vi "hardcode_libs.vi"() -> ()   [LabVIEW 2019]
uses:
  <vilib>/Utility/traverseref.llb/TRef TravTarget.ctl
  <vilib>/Utility/traverseref.llb/VI Scripting - Traverse.lvlib
panel:
  out "current":string
  out "progress":i32(slide) scale=-1.0..35.0
  # "Hardcode library paths"
  # "Use this if you have problems with DLL resolution in deployed applications. Use with caution."
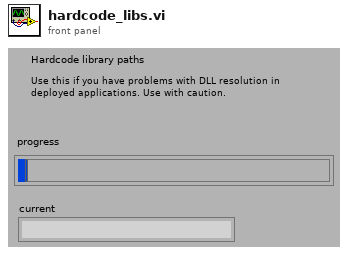
[diagram p1: front panel]
types:
  T1 = typedef "TRef TravTarget.ctl" = enum16{"FP", "BD", "Other"}
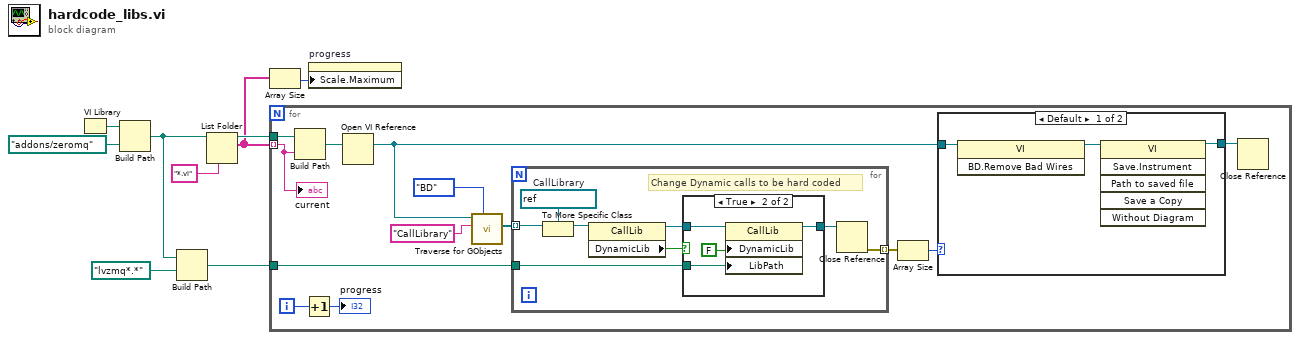
[diagram p0: block diagram]
diagram:
  n1 = VI Library() -> (path=w6:path)
  n2 = Build Path(base path=w6, name or relative path=path "addons/zeromq" ("Relative path (.)")) -> (appended path=w2:path)
  n3 = Build Path(base path=w2, name or relative path=path "lvzmq*.*" ("Library Path")) -> (appended path=w1:path)
  n4 = List Folder(path=w2, pattern="*.vi") -> (path out=w8:path, filenames=w5:string[])  [unwired: 2 in, 2 out]
  n5 = Array Size(array=w5) -> (size(s)=w4:i32)
  n6 = for {
    tunnel: w5 -> [w15] mode=indexing
    tunnel: w8 -> [w22]
    tunnel: w1 -> [w11]
    i -> [w14]
    n7 = Build Path(base path=w22, name or relative path=w15) -> (appended path=w21:path)
    n8 = Increment(x=w14) -> (x+1=→"progress":i32)
    n9 = Open VI Reference(vi path=w21) -> (vi reference=w17:refnum<vi>)  [unwired: 5 in, 1 out]
    n10 = call <vilib>:"Traverse for GObjects.vi"("Traverse Target"=TRef_TravTarget."BD", "Class Name"="CallLibrary", "VI Refnum"=w17) -> ("References"=w18:refnum<vi>[])  [unwired: 5 in, 3 out]
    n11 = for {
      tunnel: w18 -> [w34] mode=indexing
      tunnel: [w31] -> w13 mode=indexing
      tunnel: w11 -> [w30]
      w33 = refnum<vi> refnum  # CallLibrary
      # "Change Dynamic calls to be hard coded"
      n12 = To More Specific Class(target class=w33, reference=w34) -> (specific class reference=w29:refnum<vi>)  [unwired: 1 in, 1 out]
      n13 = property class="CallLib"(reference=w29) -> (reference out=w28:refnum<vi>, "DynamicLib"=w27:bool)  [unwired: 1 in, 1 out]
      n14 = case shown="True" w27 {
        tunnel: [w35 w39] -> w32
        tunnel: w30 -> [_ w37]
        tunnel: w28 -> [w35 w36]
        frame False {
        }
        frame True {
          n15 = property class="CallLib"(reference=w36, "DynamicLib"=FALSE ("Dynamic Library?"), "LibPath"=w37) -> (reference out=w39:refnum<vi>)  [unwired: 1 in, 1 out]
        }
      }
      n16 = Close Reference(reference=w32) -> (error out=w31:errorcluster)  [unwired: 1 in]
    }
    n17 = Array Size(array=w13) -> (size(s)=w12:i32)
    n18 = case shown="Default" w12 {
      tunnel: w17 -> [w24 w26]
      tunnel: [w25 w26] -> w16
      frame Default {
        n19 = invoke class="VI" method="BD.Remove Bad Wires"(reference=w24) -> (reference out=w23:refnum<vi>)  [unwired: 2 in, 2 out]
        n20 = invoke class="VI" method="Save.Instrument"(reference=w23) -> (reference out=w25:refnum<vi>)  [unwired: 5 in, 5 out]
      }
      frame 0 {
      }
    }
    n21 = Close Reference(reference=w16) -> ()  [unwired: 1 in, 1 out]
    "current" <- w15
  }
  n22 = property on="progress" class="Slide (strict)"("Scale.Maximum"=w4) -> ()  [unwired: 2 in, 2 out]
